vi "save_data_save.vi"(5 "Image":T1, 6 "Data Elements":T2(array[cluster]), 7 "Timestamp":u64, 10 "Avi Refnum":T3, 11 "Data refnum":refnum<file>) -> (0 "error out":errorcluster, 2 "Avi Refnum (duplicate)":T3, 3 "Data refnum (duplicate)":refnum<file>)   [LabVIEW 2010]
uses:
  <vilib>/vision/Avi1.llb/AviRefnum.ctl
  <vilib>/vision/Image Controls.llb/IMAQ Image.ctl
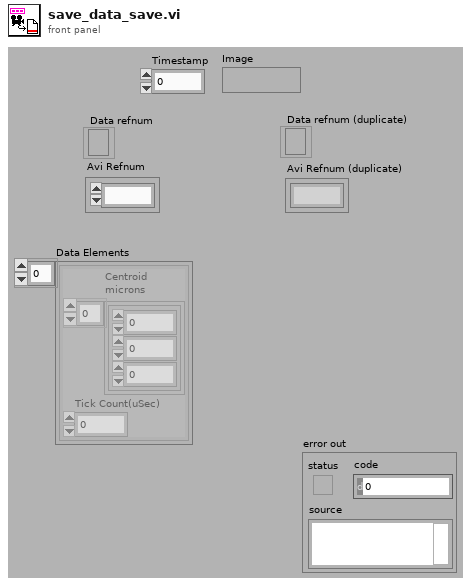
[diagram p1: front panel]
types:
  T1 = typedef "IMAQ Image.ctl" = refnum<image>
  T2 = cluster{"Centroid\nmicrons":cluster{dbl, dbl, dbl}[], "Tick Count(uSec)":dbl}[]
  T3 = typedef "AviRefnum.ctl" = refnum<k1>
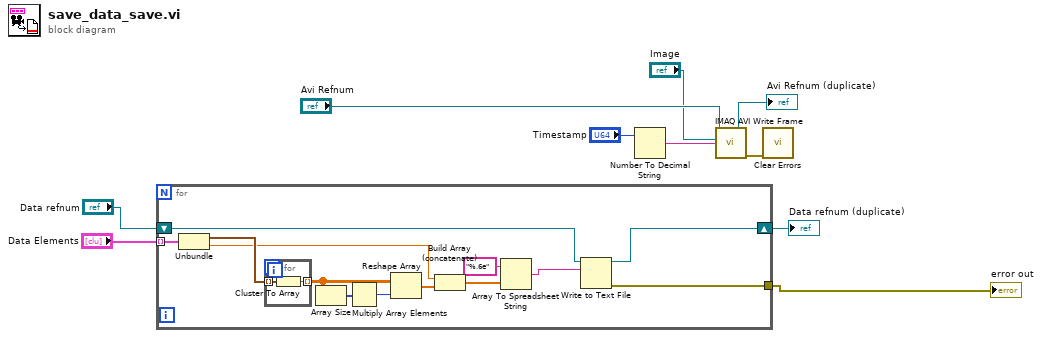
[diagram p0: block diagram]
diagram:
  n1 = for {
    tunnel: "Data Elements" -> [w23] mode=indexing
    tunnel: [w13] -> w3
    shift-right: [w11] -> w1
    shift-left: "Data refnum" -> [w12]
    n2 = Unbundle(w23) -> ("Centroid\nmicrons"=w22:cluster{dbl, dbl, dbl}[], "Tick Count(uSec)"=w17:dbl)
    n3 = for {
      tunnel: w22 -> [w25] mode=indexing
      tunnel: [w24] -> w19 mode=indexing
      n4 = Cluster To Array(cluster=w25) -> (array=w24:dbl[])
    }
    n5 = Array Size(array=w19) -> (size(s)=w20:i32[])
    n6 = Multiply Array Elements(1:w20) -> (0:w21:i32)
    n7 = Reshape Array(w19, w21) -> (w18:dbl[])
    n8 = Build Array (concatenate)(w17, w18) -> (w16:dbl[])
    n9 = Array To Spreadsheet String(array=w16, 3:"%.6e" ("format string")) -> (spreadsheet string=w14:string)  [unwired: 1 in]
    n10 = Write to Text File(file (use dialog)=w12, text=w14) -> (refnum out=w11:refnum<file>, error out=w13:errorcluster)  [unwired: 2 in, 1 out]
  }
  "error out" <- w3
  "Data refnum (duplicate)" <- w1
  n11 = Number To Decimal String(number="Timestamp") -> (decimal integer string=w8:string)  [unwired: 1 in]
  n12 = call "IMAQ AVI Write Frame"("Data"=w8, "Image"="Image", "Avi Refnum"="Avi Refnum") -> ("error out"=w4:errorcluster, "Avi Refnum (duplicate)"=→"Avi Refnum (duplicate)":T3)  [unwired: 7 in]
  n13 = call <vilib>:"Clear Errors.vi"("error in (no error)"=w4) -> ()  [unwired: 6 in, 1 out]
